vi "GetColumnData.vi"(8 "error in (no error)":errorcluster, 10 "Index":i32, 11 "AdjustableMulticolumnListbox in":refnum<class "AdjMCLB.lvclass">) -> (0 "error out":errorcluster, 2 "ColumnData":string[](array[string]), 3 "AdjustableMulticolumnListbox out":refnum<class "AdjMCLB.lvclass">)   [LabVIEW 2020, in "AdjMCLB.lvclass"]
uses:
  AdjMCLB.lvclass
  <vilib>/ErrorRing/Error Ring.xnode
  <vilib>/Utility/error.llb/Error Cluster From Error Code.vi
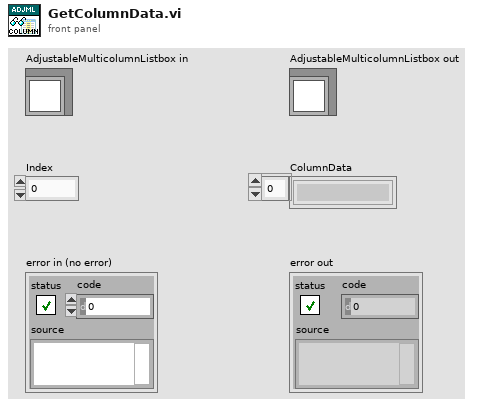
[diagram p1: front panel]
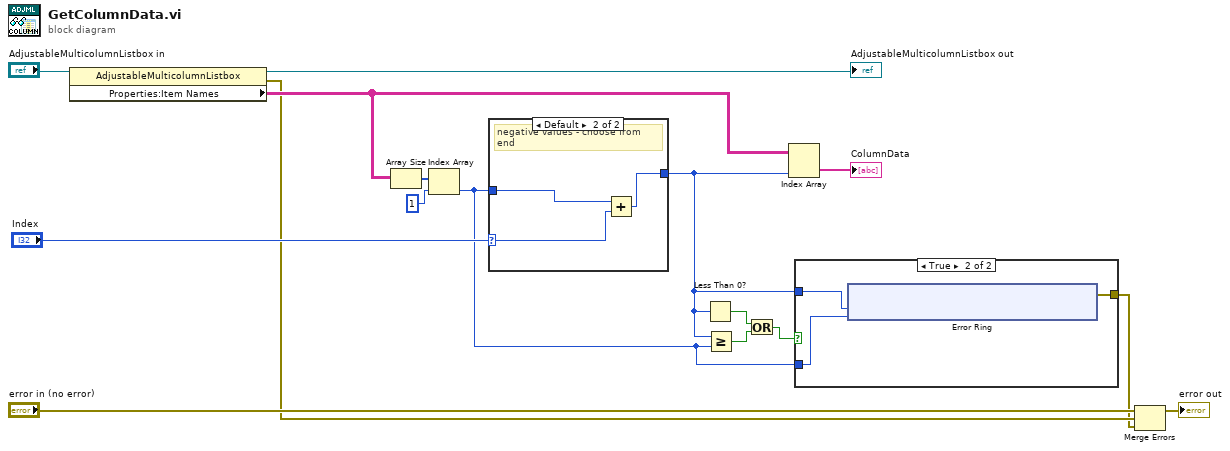
[diagram p0: block diagram]
diagram:
  n1 = property class="AdjustableMulticolumnListbox"(reference="AdjustableMulticolumnListbox in") -> (reference out=→"AdjustableMulticolumnListbox out":refnum<class "AdjMCLB.lvclass">, error out=w9:errorcluster, "Properties:Item Names"=w15:string[][])  [unwired: 1 in]
  n2 = Array Size(array=w15) -> (size(s)=w8:i32[])
  n3 = Index Array(array=w8, index=1) -> (element=w2:i32)
  n4 = case shown="Default" "Index" {
    selector: "Index" -> [w17 w19]
    tunnel: [w17 w20] -> w3
    tunnel: w2 -> [_ w18]
    frame 0.. {
    }
    frame Default {
      # "negative values - choose from end"
      n5 = Add(x=w18, y=w19) -> (x+y=w20:i32)
    }
  }
  n6 = Less Than 0?(x=w3) -> (x < 0?=w5:bool)
  n7 = Greater Or Equal?(x=w3, y=w2) -> (x >= y?=w4:bool)
  n8 = Or(x=w5, y=w4) -> (x .or. y?=w6:bool)
  n9 = Index Array(array=w15, index (col)=w3) -> (element=→"ColumnData":string[])  [unwired: 1 in]
  n10 = case shown="True" w6 {
    tunnel: w3 -> [_ w23]
    tunnel: w2 -> [_ w22]
    tunnel: [_ w21] -> w1
    frame False {
    }
    frame True {
      n11 = xnode "Error Ring"("parameter 0"=w23, "parameter 1"=w22) -> ("error out"=w21:errorcluster)
    }
  }
  n12 = Merge Errors("error in (no error)", w9, w1) -> (→"error out":errorcluster)
